vi "ShoreDefinition_2.vi"(0 "Image In":T1, 7 "error in":errorcluster) -> (20 "Image Out":T1, 27 "error out":errorcluster)   [LabVIEW 2014]
uses:
  <vilib>/vision/Image Controls.llb/IMAQ Image.ctl
  <vilib>/vision/NI_Vision_Development_Module.lvlib
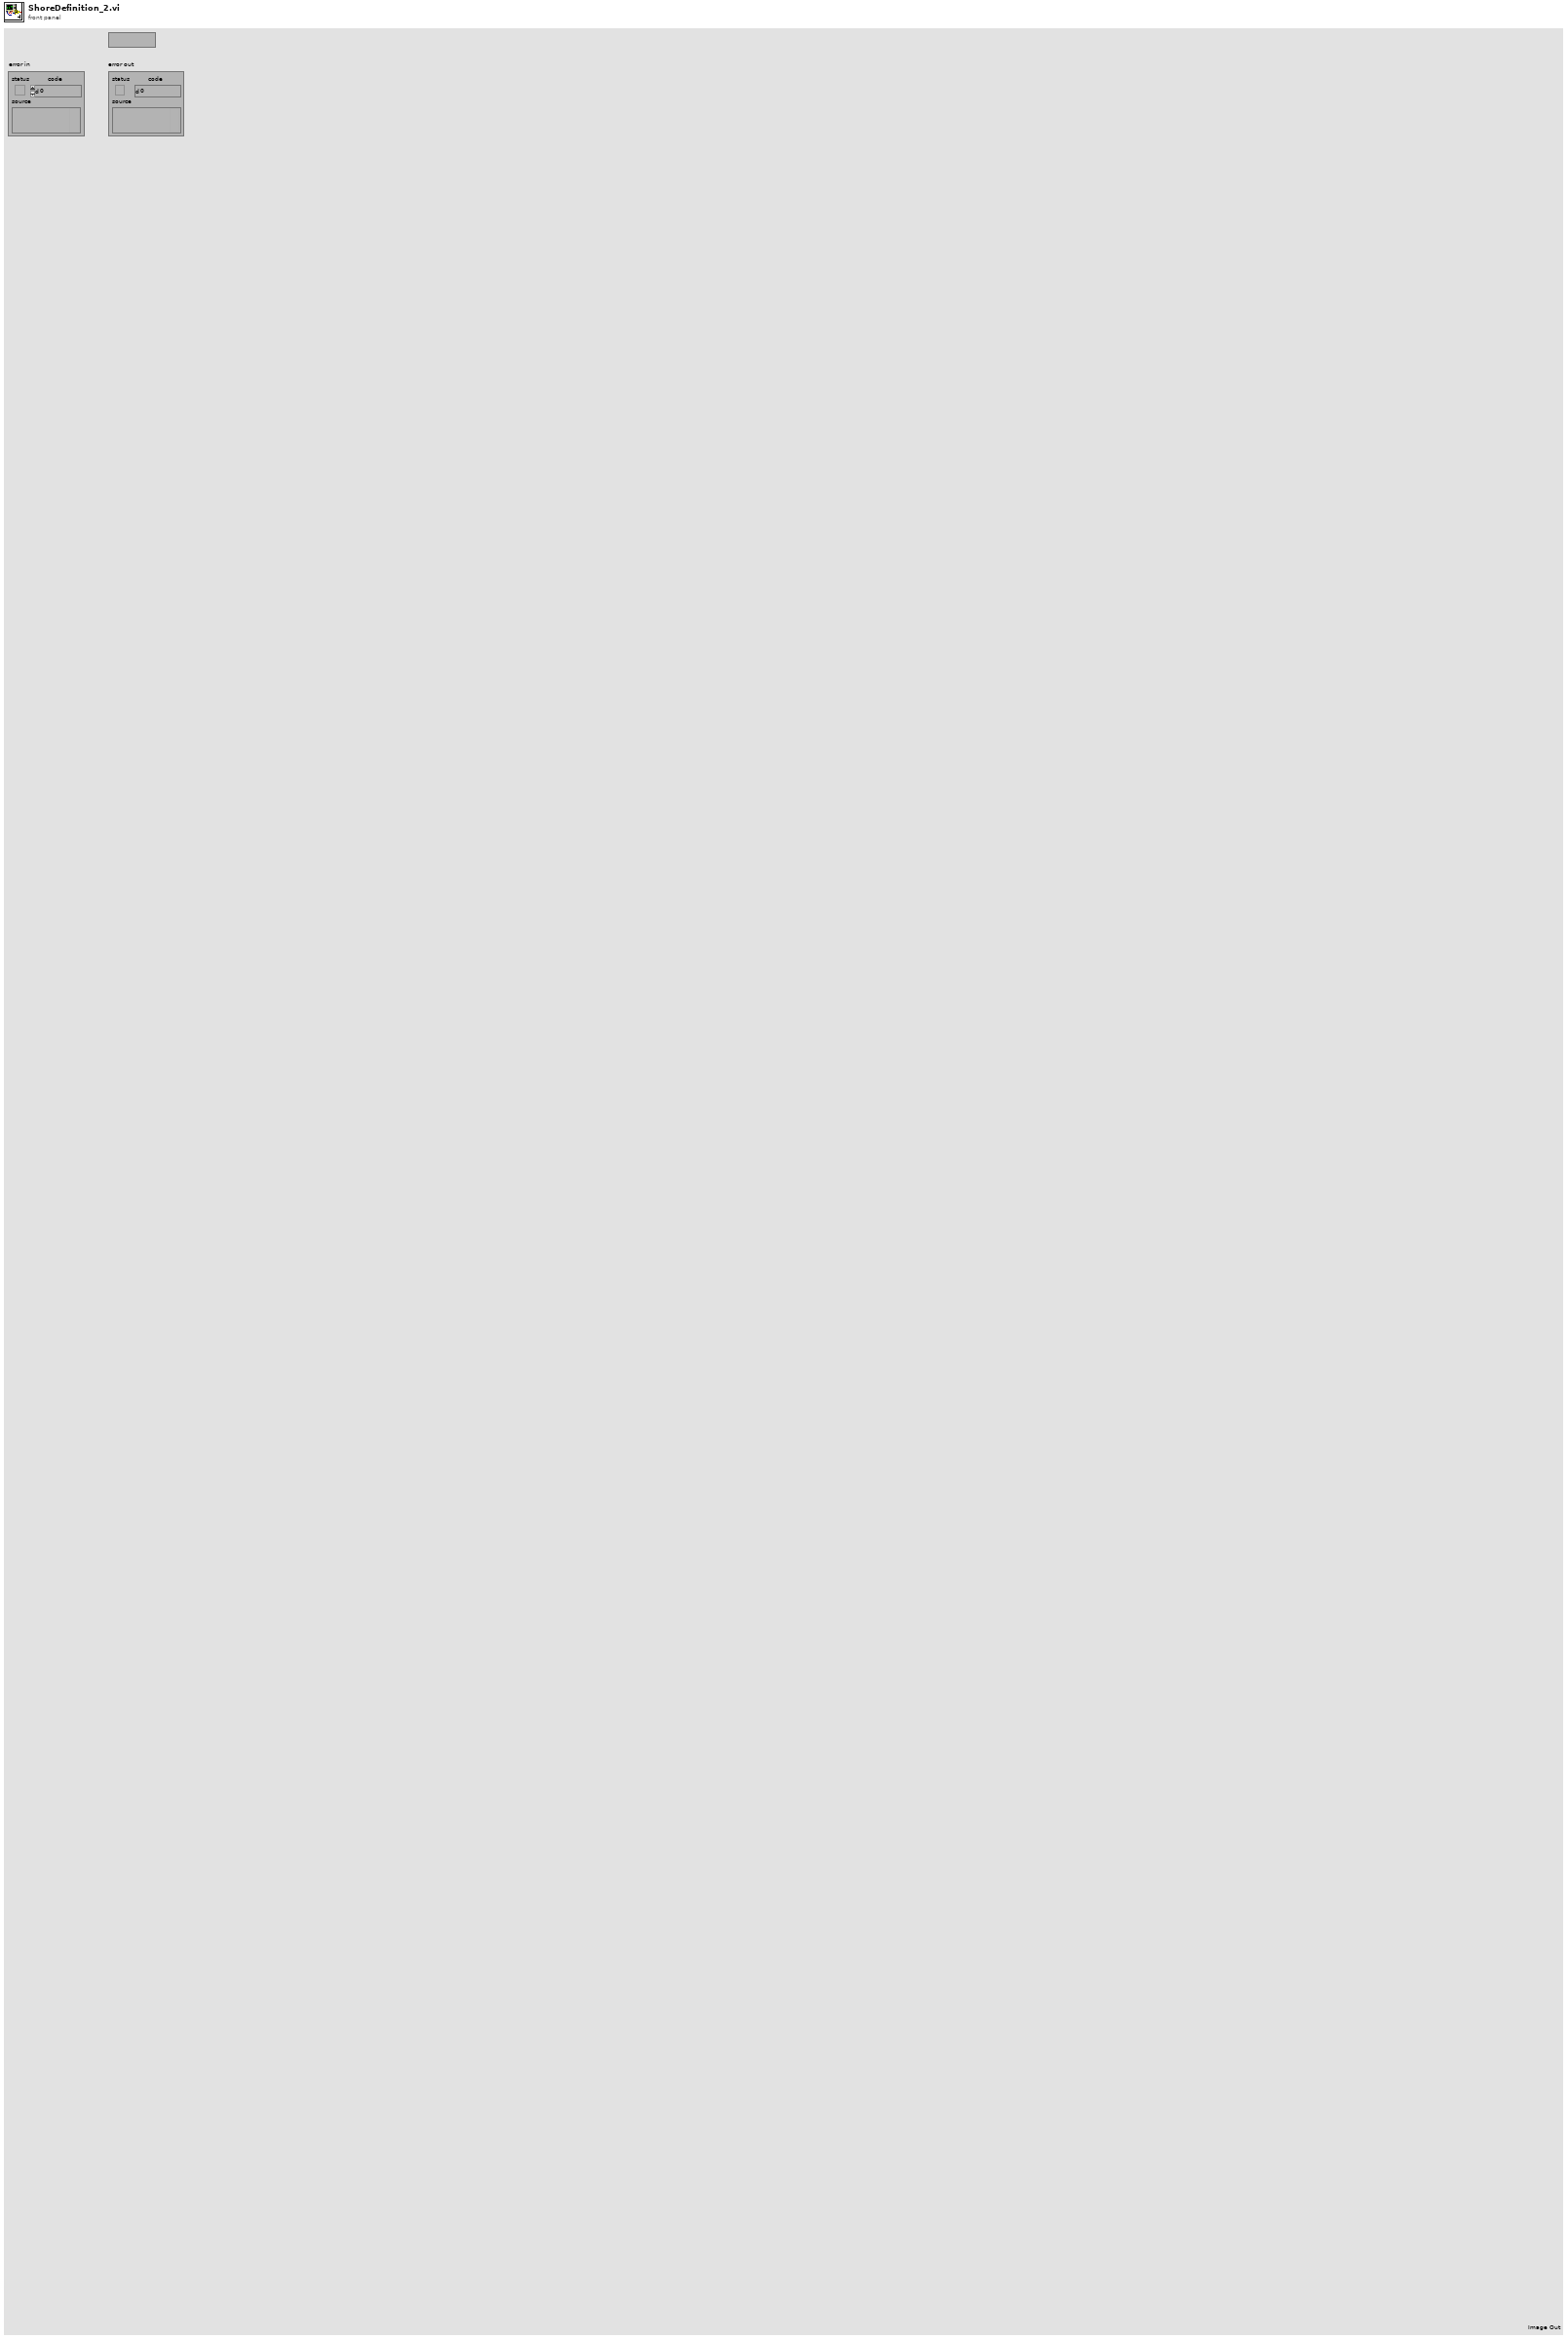
[diagram p1: front panel]
types:
  T1 = typedef "IMAQ Image.ctl" = refnum<image>
  T2 = enum32{"AutoM", "Close", "Dilate", "Erode", "Gradient", "Gradient out", "Gradient in", "Hit miss", "Open", "PClose", "POpen", "Thick", "Thin"}
  T3 = typedef "Image Type" = u32
  T4 = cluster{"Brightness":sgl, "Contrast":sgl, "Gamma":sgl}
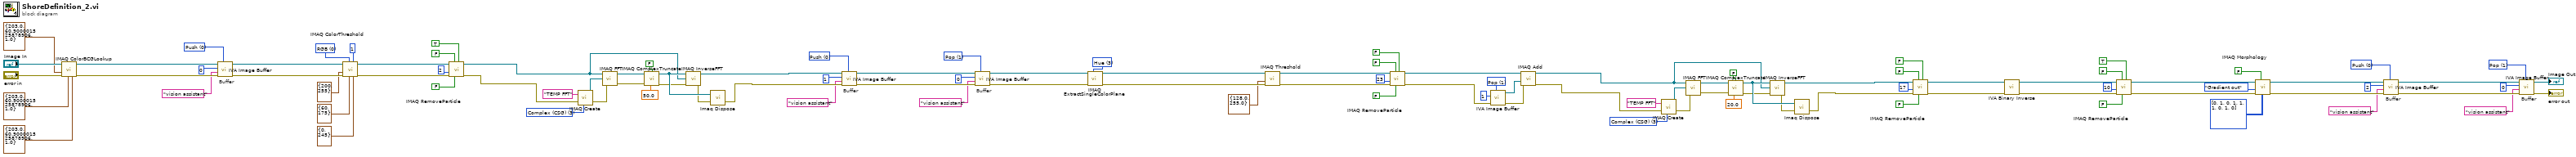
[diagram p0: block diagram]
diagram:
  w4 = u16 1 items=["Push", "Pop", "Reset"] ("Function")
  w9 = u16 0 items=["Push", "Pop", "Reset"] ("Function")
  w31 = T3 3 items=["Grayscale (U8)", "Grayscale (I16)", "Grayscale (SGL)", "Complex (CSG)", "RGB (U32)", "HSL (U32)", "RGB (U64)", "Grayscale (U16)"] ("Image Type")
  w49 = u16 1 items=["Push", "Pop", "Reset"] ("Function")
  w61 = 3 items=["Red", "Green", "Blue", "Hue", "Saturation", "Luminance", "Value", "Intensity"] ("Color Plane")
  w64 = u16 1 items=["Push", "Pop", "Reset"] ("Function")
  w69 = u16 0 items=["Push", "Pop", "Reset"] ("Function")
  w72 = T3 3 items=["Grayscale (U8)", "Grayscale (I16)", "Grayscale (SGL)", "Complex (CSG)", "RGB (U32)", "HSL (U32)", "RGB (U64)", "Grayscale (U16)"] ("Image Type")
  w96 = u16 0 items=["RGB", "HSL", "HSV", "HSI"] ("Color Mode")
  w100 = u16 0 items=["Push", "Pop", "Reset"] ("Function")
  # "Buffer"
  # "Buffer"
  # "Buffer"
  # "Buffer"
  # "Buffer"
  n1 = call "IMAQ ColorBCGLookup"("Blue BCG Values"=T4 {"Brightness"=203.0, "Contrast"=60.9, "Gamma"=1.0}, "Green BCG Values"=T4 {"Brightness"=203.0, "Contrast"=60.9, "Gamma"=1.0}, "error in (no error)"="error in", "Red BCG Values"=T4 {"Brightness"=203.0, "Contrast"=60.9, "Gamma"=1.0}, "Image Src"="Image In") -> ("error out"=w106:errorcluster, "Image Dst Out"=w102:T1)  [unwired: 2 in, 3 out]
  n2 = call <vilib>:"IVA Image Buffer.vi"("Function"=w100, "error in (no error)"=w106, "Prefix"="vision assistant", "Buffer #"=0, "Image In"=w102) -> ("error out"=w101:errorcluster, "Image Out"=w92:T1)  [unwired: 5 out]
  n3 = call "IMAQ ColorThreshold"("Blue or Luma or Val or Inten Range"=cluster{"Lower value":i32, "Upper value":i32} {"Lower value"=0, "Upper value"=245}, "Replace Value"=1, "Green or Sat Range"=cluster{"Lower value":i32, "Upper value":i32} {"Lower value"=60, "Upper value"=175}, "Color Mode"=w96, "error in (no error)"=w101, "Red or Hue Range"=cluster{"Lower value":i32, "Upper value":i32} {"Lower value"=200, "Upper value"=255}, "Image Src"=w92) -> ("error out"=w91:errorcluster, "Image Dst Out"=w86:T1)  [unwired: 1 in, 2 out]
  n4 = call "IMAQ RemoveParticle"("Connectivity 4/8 (8)"=TRUE, "Low Pass/High Pass (Low)"=FALSE, "Square/Hexa (Square)"=FALSE, "error in (no error)"=w91, "Number of Erosion"=2, "Image Src"=w86) -> ("error out"=w85:errorcluster, "Image Dst Out"=w75:T1)  [unwired: 1 in, 3 out]
  n5 = call "IMAQ Create"("Image Name"="TEMP FFT", "Image Type"=w72, "error in (no error)"=w85) -> ("New Image"=w83:T1, "error out"=w76:errorcluster)  [unwired: 1 in, 1 out]
  n6 = call "IMAQ FFT"("error in (no error)"=w76, "Image Dst"=w83, "Image Src"=w75) -> ("error out"=w81:errorcluster, "Image Dst Out"=w82:T1)  [unwired: 1 out]
  n7 = call "IMAQ ComplexTruncate"("error in (no error)"=w81, "Truncation Frequency %"=sgl 50.0, "Image Src"=w82, "Low pass/High pass (Low pass)"=FALSE) -> ("error out"=w79:errorcluster, "Image Dst Out"=w80:T1)  [unwired: 1 in, 2 out]
  n8 = call "IMAQ InverseFFT"("error in (no error)"=w79, "Image Dst"=w75, "Image Src"=w80) -> ("error out"=w78:errorcluster, "Image Dst Out"=w71:T1)  [unwired: 1 out]
  n9 = call "Imaq Dispose"("Image"=w80, "error in (no error)"=w78) -> ("error out"=w77:errorcluster)  [unwired: 1 in, 3 out]
  n10 = call <vilib>:"IVA Image Buffer.vi"("Function"=w69, "error in (no error)"=w77, "Prefix"="vision assistant", "Buffer #"=1, "Image In"=w71) -> ("error out"=w70:errorcluster, "Image Out"=w66:T1)  [unwired: 5 out]
  n11 = call <vilib>:"IVA Image Buffer.vi"("Function"=w64, "error in (no error)"=w70, "Prefix"="vision assistant", "Buffer #"=0, "Image In"=w66) -> ("error out"=w65:errorcluster, "Image Out"=w60:T1)  [unwired: 5 out]
  n12 = call "IMAQ ExtractSingleColorPlane"("Color Plane"=w61, "error in (no error)"=w65, "Image Src"=w60) -> ("error out"=w59:errorcluster, "Image Dst Out"=w57:T1)  [unwired: 1 in, 6 out]
  n13 = call "IMAQ Threshold"("error in (no error)"=w59, "Range"=cluster{"Lower value":sgl, "Upper value":sgl} {"Lower value"=128.0, "Upper value"=255.0}, "Image Src"=w57) -> ("error out"=w56:errorcluster, "Image Dst Out"=w51:T1)  [unwired: 3 in, 4 out]
  n14 = call "IMAQ RemoveParticle"("Connectivity 4/8 (8)"=FALSE, "Low Pass/High Pass (Low)"=FALSE, "Square/Hexa (Square)"=FALSE, "error in (no error)"=w56, "Number of Erosion"=23, "Image Src"=w51) -> ("error out"=w50:errorcluster, "Image Dst Out"=w46:T1)  [unwired: 1 in, 3 out]
  n15 = call <vilib>:"IVA Image Buffer.vi"("Function"=w49, "error in (no error)"=w50, "Buffer #"=1) -> ("error out"=w45:errorcluster, "Image Out"=w47:T1)  [unwired: 2 in, 5 out]
  n16 = call "IMAQ Add"("Image Src A"=w46, "Image Src B"=w47, "error in (no error)"=w45) -> ("Image Dst Out"=w34:T1, "error out"=w44:errorcluster)  [unwired: 2 in, 2 out]
  n17 = call "IMAQ Create"("Image Name"="TEMP FFT", "Image Type"=w31, "error in (no error)"=w44) -> ("New Image"=w42:T1, "error out"=w35:errorcluster)  [unwired: 1 in, 1 out]
  n18 = call "IMAQ FFT"("error in (no error)"=w35, "Image Dst"=w42, "Image Src"=w34) -> ("error out"=w40:errorcluster, "Image Dst Out"=w41:T1)  [unwired: 1 out]
  n19 = call "IMAQ ComplexTruncate"("error in (no error)"=w40, "Truncation Frequency %"=sgl 20.0, "Image Src"=w41, "Low pass/High pass (Low pass)"=FALSE) -> ("error out"=w38:errorcluster, "Image Dst Out"=w39:T1)  [unwired: 1 in, 2 out]
  n20 = call "IMAQ InverseFFT"("error in (no error)"=w38, "Image Dst"=w34, "Image Src"=w39) -> ("error out"=w37:errorcluster, "Image Dst Out"=w26:T1)  [unwired: 1 out]
  n21 = call "Imaq Dispose"("Image"=w39, "error in (no error)"=w37) -> ("error out"=w36:errorcluster)  [unwired: 1 in, 3 out]
  n22 = call "IMAQ RemoveParticle"("Connectivity 4/8 (8)"=FALSE, "Low Pass/High Pass (Low)"=FALSE, "Square/Hexa (Square)"=FALSE, "error in (no error)"=w36, "Number of Erosion"=17, "Image Src"=w26) -> ("error out"=w25:errorcluster, "Image Dst Out"=w24:T1)  [unwired: 1 in, 3 out]
  n23 = call <vilib>:"IVA Binary Inverse.vi"("error in (no error)"=w25, "Image In"=w24) -> ("error out"=w23:errorcluster, "Image Out"=w18:T1)  [unwired: 8 out]
  n24 = call "IMAQ RemoveParticle"("Connectivity 4/8 (8)"=TRUE, "Low Pass/High Pass (Low)"=FALSE, "Square/Hexa (Square)"=FALSE, "error in (no error)"=w23, "Number of Erosion"=10, "Image Src"=w18) -> ("error out"=w17:errorcluster, "Image Dst Out"=w13:T1)  [unwired: 1 in, 3 out]
  n25 = call "IMAQ Morphology"("Structuring Element"=i32[][] [[0, 1, 0], [1, 1, 1], [0, 1, 0]], "Square/Hexa (Square)"=FALSE, "error in (no error)"=w17, "Operation"=T2."Gradient out", "Image Src"=w13) -> ("error out"=w12:errorcluster, "Image Dst Out"=w11:T1)  [unwired: 2 in, 3 out]
  n26 = call <vilib>:"IVA Image Buffer.vi"("Function"=w9, "error in (no error)"=w12, "Prefix"="vision assistant", "Buffer #"=2, "Image In"=w11) -> ("error out"=w10:errorcluster, "Image Out"=w6:T1)  [unwired: 5 out]
  n27 = call <vilib>:"IVA Image Buffer.vi"("Function"=w4, "error in (no error)"=w10, "Prefix"="vision assistant", "Buffer #"=0, "Image In"=w6) -> ("error out"=→"error out":errorcluster, "Image Out"=→"Image Out":T1)  [unwired: 5 out]
